vi "Notify Daemon Stopped.vi"(8 "error in (no error)":errorcluster, 11 "Network Slave in":refnum<class "Network Slave.lvclass">) -> (0 "error out":errorcluster, 3 "Network Slave out":refnum<class "Network Slave.lvclass">)   [LabVIEW 2017, in "SubVIs.lvlib" / "Network Slave.lvclass"]
uses:
  <vilib>/Modbus/subvis/Protocol/Interfaces/Network Slave/Network Slave.lvclass
  <vilib>/Modbus/subvis/Protocol/Interfaces/Network Slave/Network Slave.lvclass/Network Slave.ctl
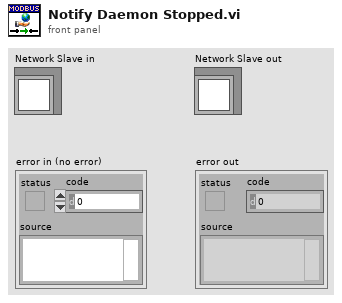
[diagram p1: front panel]
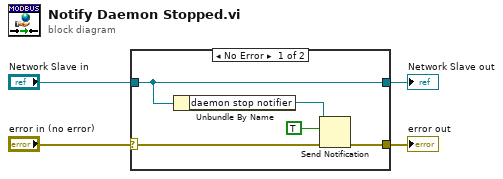
[diagram p0: block diagram]
diagram:
  n1 = case shown="No Error" "error in (no error)" {
    selector: "error in (no error)" -> [w6 w11]
    tunnel: [w5 w11] -> w3
    tunnel: [w9 w10] -> w1
    tunnel: "Network Slave in" -> [w9 w10]
    frame No Error {
      n2 = Unbundle By Name(w9) -> ("daemon stop notifier"=w8:refnum<notifier>)
      n3 = Send Notification(notification=TRUE, notifier=w8, error in (no error)=w6) -> (error out=w5:errorcluster)  [unwired: 1 out]
    }
    frame Error {
    }
  }
  "error out" <- w3
  "Network Slave out" <- w1
